vi "main--material example.vi"() -> ()   [LabVIEW 2021]
doc: "Example UI VI -- shows a couple example buttons and how to use the load and application VIs to theme the sample UI\n\n<b>Code Developed By:</b>\nTechnology Service Corporation\nwww.tsc.com/atcs\n\nDeveloper:\nDaniel Coons"
uses:
  Material Theme/Material Theme.lvclass
  user32.dll
panel:
  in  "tab control--Inverse Primary":enum32{"Page 1", "Page 2"}(tab)
  in  "File Path (theme)":path
  in  "theme-switch":bool
  out "status":string
  in  "filled--text--rectangular":bool
  in  "tonal--icons--rounded":bool
  in  "outline--text--rectangular":bool
  in  "FAB Button":bool
  in  "Close":bool
  out "header":bool
  # "control UI role = Secondary"
  # "Note:  run the VI to see dynamic theme in action!"
  # "Front Panel Rule: Surface"
  # "control UI role = Primary"
  # "control UI role = Primary"
  # "Decoration--Surface Container Low"
  # "control UI role = Tertiary"
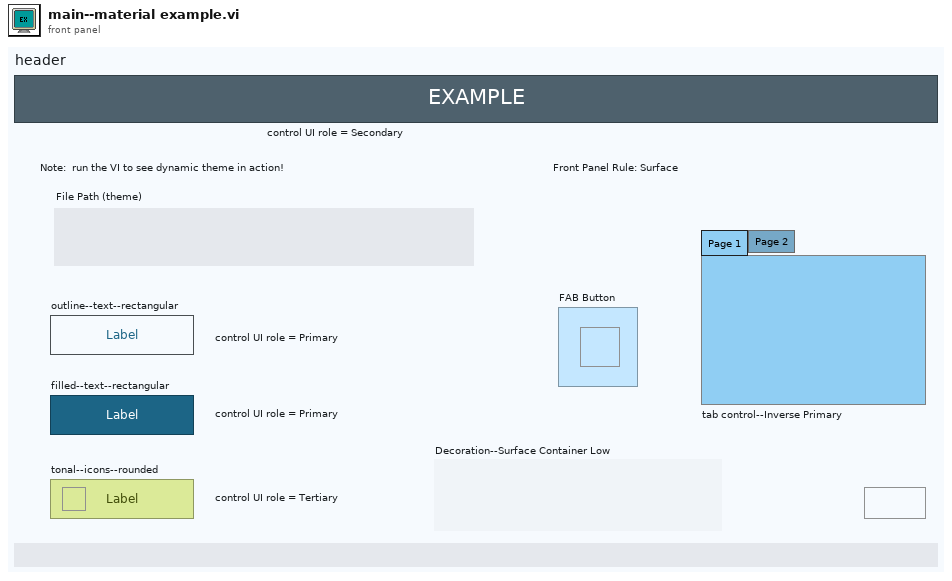
[diagram p1: front panel]
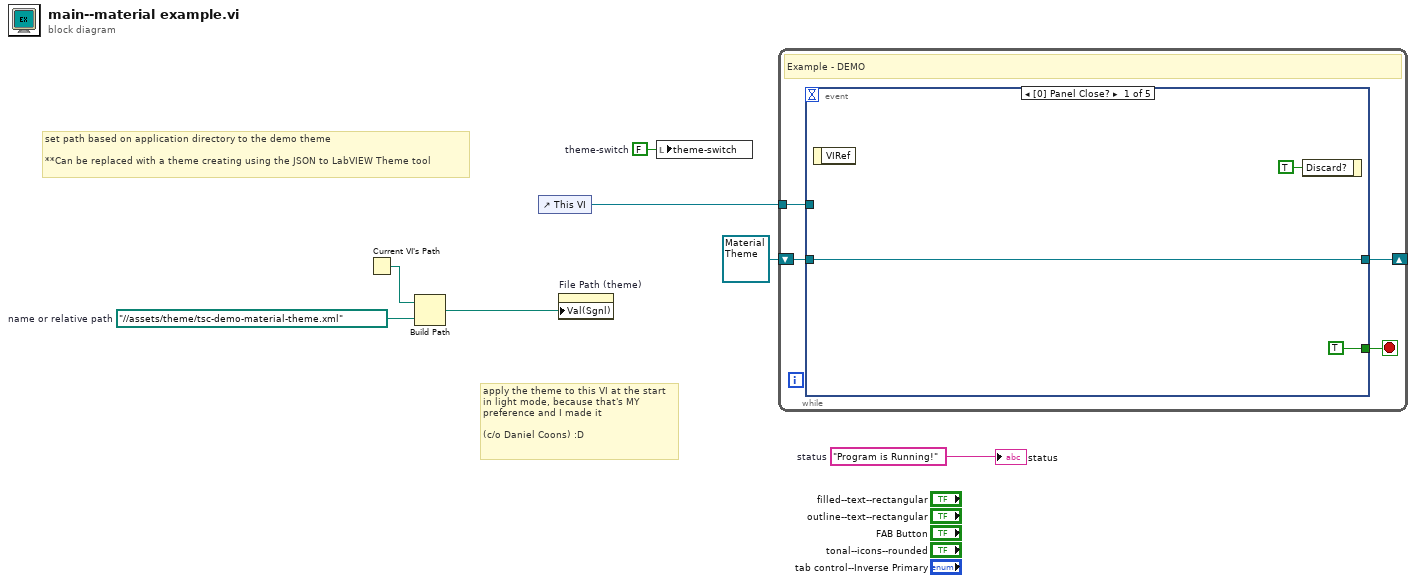
[diagram p0: block diagram]
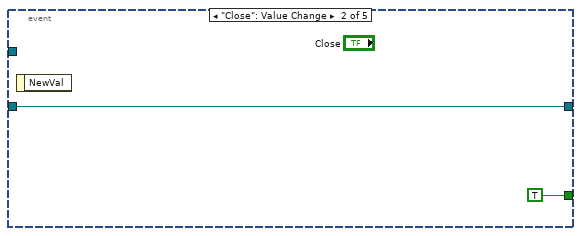
[diagram p2: hidden frame]
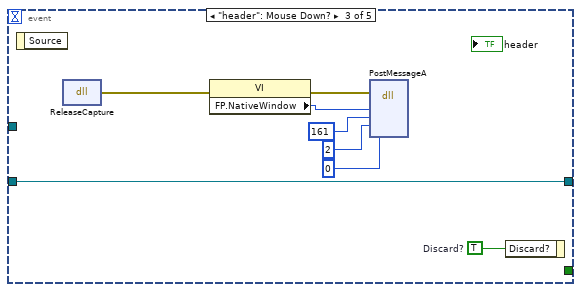
[diagram p3: hidden frame]
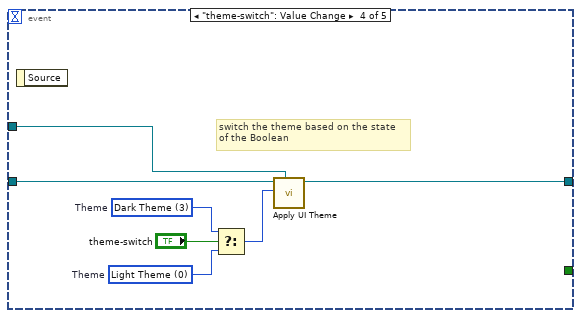
[diagram p4: hidden frame]
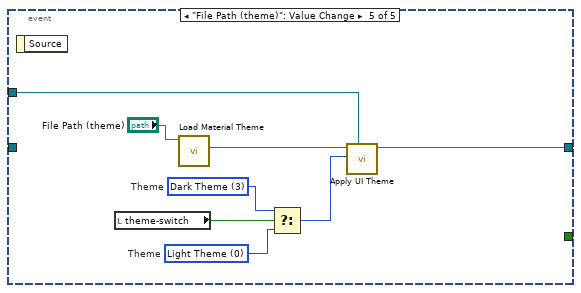
[diagram p5: hidden frame]
diagram:
  w3 = FALSE  # theme-switch
  w5 = path "../../assets/theme/tsc-demo-material-theme.xml"  # name or relative path
  w7 = "Program is Running!"  # status
  # "apply the theme to this VI at the start\nin light mode, because that's MY \npreference and I made it\n\n(c/o Daniel Coons) :D"
  # "set path based on application directory to the demo theme\n\n**Can be replaced with a theme creating using the JSON to LabVIEW Theme tool"
  n1 = Current VI's Path() -> (path=w6:path)
  n2 = Build Path(base path=w6, name or relative path=w5) -> (appended path=w2:path)
  n3 = control-ref of="This VI"() -> (w4:refnum<vi>)
  n4 = property on="File Path (theme)" class="Path"("Val(Sgnl)"=w2) -> ()  [unwired: 2 in, 2 out]
  n5 = local write "theme-switch"(w3) -> ()
  n6 = while {
    tunnel: w4 -> [w9]
    shift-right: [w8] -> _
    shift-left: refnum<class "Material Theme.lvclass"> refnum ("Material Theme out") -> [w10]
    stop <- w11 stop-if-true
    # "Example - DEMO"
    n7 = event shown="[0] Panel Close?" {
      selector: _ -> [_ _ _ _ _]
      dyn-events: _ -> [_ _ _ _ _]
      timeout: _ -> [_ _ _ _ _]
      tunnel: [TRUE TRUE _ _ _] -> w11
      tunnel: w10 -> [w12 w15 w17 w31 _]
      tunnel: w9 -> [_ _ _ w30 w36]
      tunnel: [w12 w15 w17 w25 w37] -> w8
      event Panel Close? {
        n8 = event-data() -> ()  [unwired: 1 in, 1 out]
        n9 = event-data("Discard?"=TRUE) -> ()  [unwired: 1 in, 1 out]
      }
      event "Close": Value Change {
        n10 = event-data() -> ()  [unwired: 1 in, 1 out]
      }
      event "header": Mouse Down? {
        w24 = TRUE  # Discard?
        n11 = event-data() -> ()  [unwired: 1 in, 1 out]
        n12 = dll-call lib="user32.dll" fn="ReleaseCapture"() -> (error out=w20:errorcluster)  [unwired: 4 in, 1 out]
        n13 = property class="VI"(error in=w20) -> (error out=w19:errorcluster, "FP.NativeWindow"=w18:u64)  [unwired: 1 in, 1 out]
        n14 = dll-call lib="user32.dll" fn="PostMessageA"(error in=w19, "hWnd"=w18, "Msg"=161, "wParam"=2, "lParam"=0) -> ()  [unwired: 7 in, 2 out]
        n15 = event-data("Discard?"=w24) -> ()  [unwired: 1 in, 1 out]
      }
      event "theme-switch": Value Change {
        w28 = u16 3 items=["Light Theme", "Light Medium Contrast", "Light High Contrast", "Dark Theme", "Dark Medium Contrast", "Dark High Constrast"]  # Theme
        w27 = u16 0 items=["Light Theme", "Light Medium Contrast", "Light High Contrast", "Dark Theme", "Dark Medium Contrast", "Dark High Constrast"]  # Theme
        # "switch the theme based on the state\nof the Boolean"
        n16 = event-data() -> ()  [unwired: 1 in, 1 out]
        n17 = Select(t=w28, s="theme-switch", f=w27) -> (s? t:f=w26:u16)
        n18 = call "Apply UI Theme.vi"("VI Refnum"=w30, "Theme Mode"=w26, "Material Theme in"=w31) -> ("Material Theme out"=w25:refnum<class "Material Theme.lvclass">)  [unwired: 7 in, 1 out]
      }
      event "File Path (theme)": Value Change {
        w33 = u16 3 items=["Light Theme", "Light Medium Contrast", "Light High Contrast", "Dark Theme", "Dark Medium Contrast", "Dark High Constrast"]  # Theme
        w34 = u16 0 items=["Light Theme", "Light Medium Contrast", "Light High Contrast", "Dark Theme", "Dark Medium Contrast", "Dark High Constrast"]  # Theme
        n19 = event-data() -> ()  [unwired: 1 in, 1 out]
        n20 = local read "theme-switch"() -> (w35:bool)
        n21 = call "Load Material Theme.vi"("file path (use dialog)"="File Path (theme)") -> ("Theme"=w39:refnum<class "Material Theme.lvclass">)  [unwired: 9 in, 1 out]
        n22 = Select(t=w33, s=w35, f=w34) -> (s? t:f=w32:u16)
        n23 = call "Apply UI Theme.vi"("VI Refnum"=w36, "Theme Mode"=w32, "Material Theme in"=w39) -> ("Material Theme out"=w37:refnum<class "Material Theme.lvclass">)  [unwired: 7 in, 1 out]
      }
    }
  }
  "status" <- w7
